vi "Swap X and Y.vi"   [LabVIEW 2019, in "xy_utilities.lvlib"]
doc: "Swap the x and y arrays.\n\nWire data to the data input to determine the polymorphic instance to use or manually select the instance."
uses:
  xy_utilities.lvlib
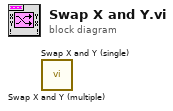
[diagram p0: block diagram]
diagram:
  n1 = call "Swap X and Y (multiple).vi"() -> ()  [unwired: 10 in, 2 out]
  n2 = call "Swap X and Y (single).vi"() -> ()  [unwired: 10 in, 2 out]
